vi "RIGOLburstsetup.vi"(8 "Ncycles":u16, 9 "Phase (degrees 0-360)":dbl, 10 "Amplitude (Vpp)":dbl, 11 "Frequency (MHz)":dbl) -> ()   [LabVIEW 2009]
panel:
  out "read buffer":string
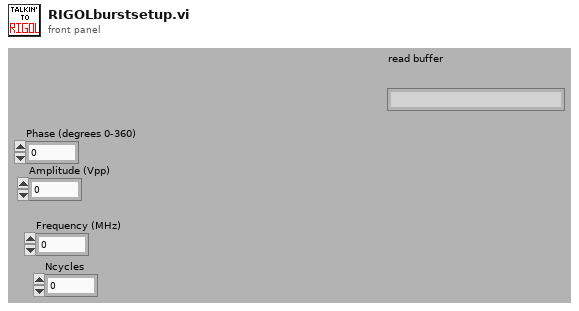
[diagram p1: front panel]
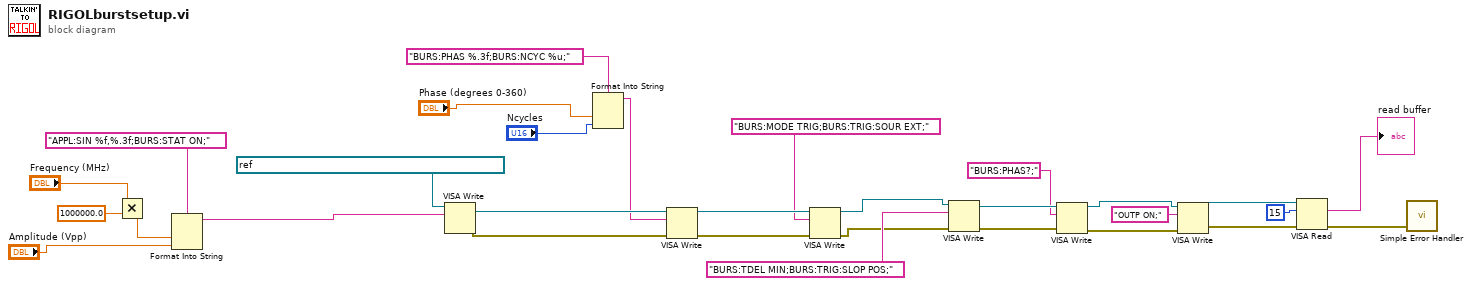
[diagram p0: block diagram]
diagram:
  n1 = Multiply(x="Frequency (MHz)", y=1000000.0) -> (x*y=w26:dbl)
  n2 = Format Into String(format string="APPL:SIN %f,%.3f;BURS:STAT ON;", w26, "Amplitude (Vpp)") -> (resulting string=w24:string)  [unwired: 2 in, 1 out]
  n3 = VISA Write(VISA resource name=refnum<visa-resource-name> "USB0::0x1AB1::0x0641::DG4B142100247::INSTR", write buffer=w24) -> (VISA resource name out=w23:refnum<visa-resource-name>, error out=w22:errorcluster)  [unwired: 1 in, 1 out]
  n4 = Format Into String(format string="BURS:PHAS %.3f;BURS:NCYC %u;" ("write buffer"), "Phase (degrees 0-360)", "Ncycles") -> (resulting string=w20:string)  [unwired: 2 in, 1 out]
  n5 = VISA Write(VISA resource name=w23, write buffer=w20, error in (no error)=w22) -> (VISA resource name out=w19:refnum<visa-resource-name>, error out=w18:errorcluster)  [unwired: 1 out]
  n6 = VISA Write(VISA resource name=w19, write buffer="BURS:MODE TRIG;BURS:TRIG:SOUR EXT;", error in (no error)=w18) -> (VISA resource name out=w10:refnum<visa-resource-name>, error out=w9:errorcluster)  [unwired: 1 out]
  n7 = VISA Write(VISA resource name=w10, write buffer="BURS:TDEL MIN;BURS:TRIG:SLOP POS;", error in (no error)=w9) -> (VISA resource name out=w3:refnum<visa-resource-name>, error out=w2:errorcluster)  [unwired: 1 out]
  n8 = VISA Write(VISA resource name=w3, write buffer="BURS:PHAS?;", error in (no error)=w2) -> (VISA resource name out=w5:refnum<visa-resource-name>, error out=w4:errorcluster)  [unwired: 1 out]
  n9 = VISA Write(VISA resource name=w5, write buffer="OUTP ON;", error in (no error)=w4) -> (VISA resource name out=w13:refnum<visa-resource-name>, error out=w12:errorcluster)  [unwired: 1 out]
  n10 = VISA Read(VISA resource name=w13, byte count=u32 15, error in (no error)=w12) -> (read buffer=→"read buffer":string, error out=w8:errorcluster)  [unwired: 2 out]
  n11 = call <vilib>:"Simple Error Handler.vi"("error in (no error)"=w8) -> ()  [unwired: 4 in, 5 out]
